vi "Remove empty data rows.vi"(9 "Array In":string[][](array[string])) -> (1 "Array Out":string[][](array[string]))   [LabVIEW 2013]
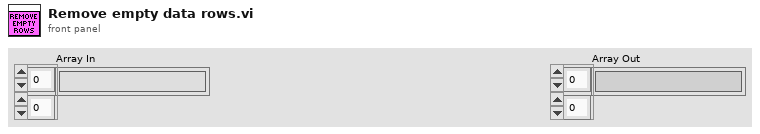
[diagram p1: front panel]
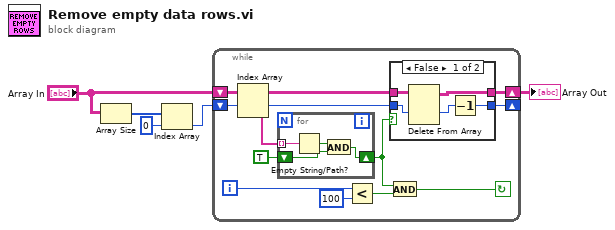
[diagram p0: block diagram]
diagram:
  n1 = Array Size(array="Array In") -> (size(s)=w5:i32[])
  n2 = Index Array(array=w5, index=0) -> (element=w2:i32)
  n3 = while {
    shift-right: [w13] -> w1
    shift-left: "Array In" -> [w14]
    shift-right: [w11] -> _
    shift-left: w2 -> [w12]
    i -> [w10]
    stop <- w6 continue-if-true
    n4 = Index Array(array=w14, index (row)=w12) -> (element=w16:string[])  [unwired: 1 in]
    n5 = for {
      tunnel: w16 -> [w26] mode=indexing
      shift-right: [w24] -> w7
      shift-left: TRUE -> [w23]
      n6 = Empty String/Path?(string/path=w26) -> (empty?=w25:bool)
      n7 = And(x=w25, y=w23) -> (x .and. y?=w24:bool)
    }
    n8 = Less?(x=w10, y=100) -> (x < y?=w8:bool)
    n9 = case shown="False" w7 {
      tunnel: w14 -> [w20 w22]
      tunnel: [w19 w22] -> w13
      tunnel: w12 -> [w18 w21]
      tunnel: [w17 w21] -> w11
      frame False {
        n10 = Delete From Array(array=w20, index (row)=w18) -> (array with subset deleted=w19:string[][])  [unwired: 2 in, 1 out]
        n11 = Decrement(x=w18) -> (x-1=w17:i32)
      }
      frame True {
      }
    }
    n12 = And(x=w7, y=w8) -> (x .and. y?=w6:bool)
  }
  "Array Out" <- w1
